vi "ziGetEventTriggerSample.vi"(8 "Error In":errorcluster, 10 "Trigger Sample In":T1, 11 "Handle In":T2 {"Handle" format="0x%08x"; "Conn" format="0x%08x"}) -> (0 "Error Out":errorcluster, 2 "Trigger Sample Out":T1, 3 "Handle Out":T2 {"Handle" format="0x%08x"; "Conn" format="0x%08x"})   [LabVIEW 2018, in "Zurich Instruments LabOne.lvlib"]
uses:
  Zurich Instruments LabOne.lvlib
  <instrlib>/Zurich Instruments LabOne/Private/ziLV64.framework
  ziTypeHandle.ctl
  ziTypeTriggerSample.ctl
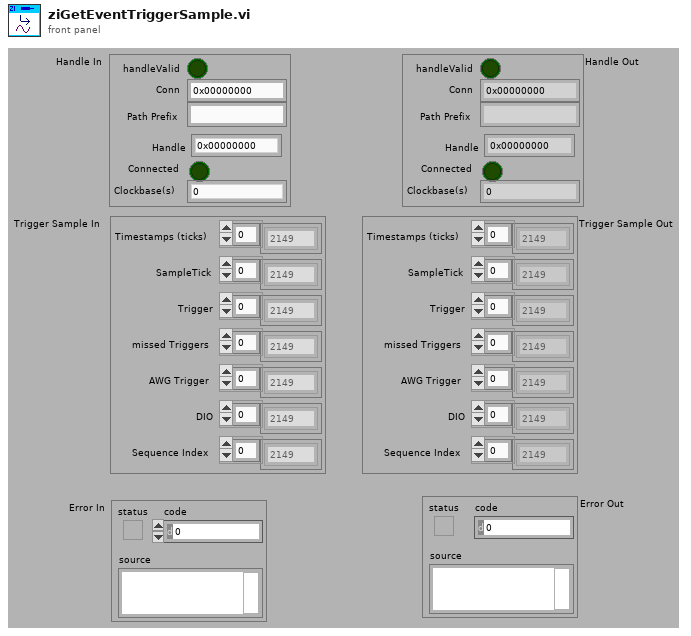
[diagram p1: front panel]
types:
  T1 = typedef "Zurich Instruments LabOne.lvlib/ziTypeTriggerSample.ctl" = cluster{"timeStamp":u64[], "sampleTick":u64[], "trigger":u32[], "missedTriggers":u32[], "awgTrigger":u32[], "dio":u32[], "sequenceIndex":u32[]}
  T2 = typedef "Zurich Instruments LabOne.lvlib/ziTypeHandle.ctl" = cluster{"handleValid":bool, "Conn":u64, "Path Prefix":string, "Handle":u64, "Connected":bool, "Clockbase(s)":dbl}
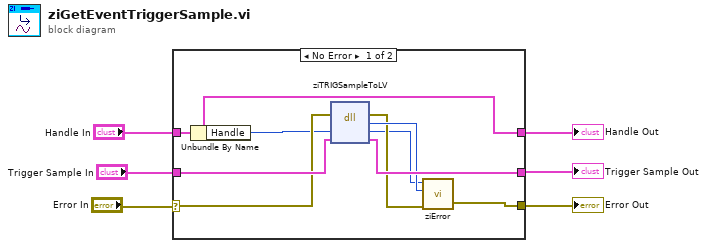
[diagram p0: block diagram]
diagram:
  n1 = case shown="No Error" "Error In" {
    selector: "Error In" -> [w12 w16]
    tunnel: "Handle In" -> [w8 w18]
    tunnel: [w8 w18] -> w5
    tunnel: [w15 w17] -> w2
    tunnel: "Trigger Sample In" -> [w14 w17]
    tunnel: [w13 w16] -> w4
    frame No Error {
      n2 = Unbundle By Name(w8) -> ("Handle"=w11:u64)
      n3 = dll-call lib="Applications/National Instruments/LabVIEW 2019 64-bit/instr.lib/Zurich Instruments LabOne/Private/ziLV*.*" fn="ziTRIGSampleToLV"(error in=w12, "ziEventBuffer"=w11, "DemodSample"=w14) -> (error out=w9:errorcluster, "return type"=w10:u32, "ziEventBuffer"=w7:u64, "DemodSample"=w15:T1)  [unwired: 2 in, 1 out]
      n4 = call "ziError.vi"("Conn"=w7, "ziErrorCode"=w10, "Error In"=w9) -> ("Error Out"=w13:errorcluster)  [unwired: 2 in, 1 out]
    }
    frame Error {
    }
  }
  "Handle Out" <- w5
  "Error Out" <- w4
  "Trigger Sample Out" <- w2
